vi "add.issue.vi"(0 "issues in":map{i32, T2}(c390), 1 "creator map in":T1(c390), 2 "Path":path, 5 "char map in":T3, 7 "concept map in":T3, 9 "story map in":T3, 11 "error in (no error)":errorcluster, 12 "team map in":T3) -> (3 "creator map out":T1(c390), 4 "issues out":map{i32, T2}(c390), 6 "char map out":T3, 8 "concept map out":T3, 10 "story map out":T3, 14 "team map out":T3, 15 "error out":errorcluster)   [LabVIEW 2024, in "manager_daemon.lvclass"]
uses:
  manager_daemon.lvclass
  type_defs/sub-map--map.ctl
  type_defs/SubData--cluster.ctl
  type_defs/IssueData--clustrer.ctl
  manager_daemon.lvclass/manager_daemon.ctl
  CV_Shared_Library/CV_Shared_Library.lvlib
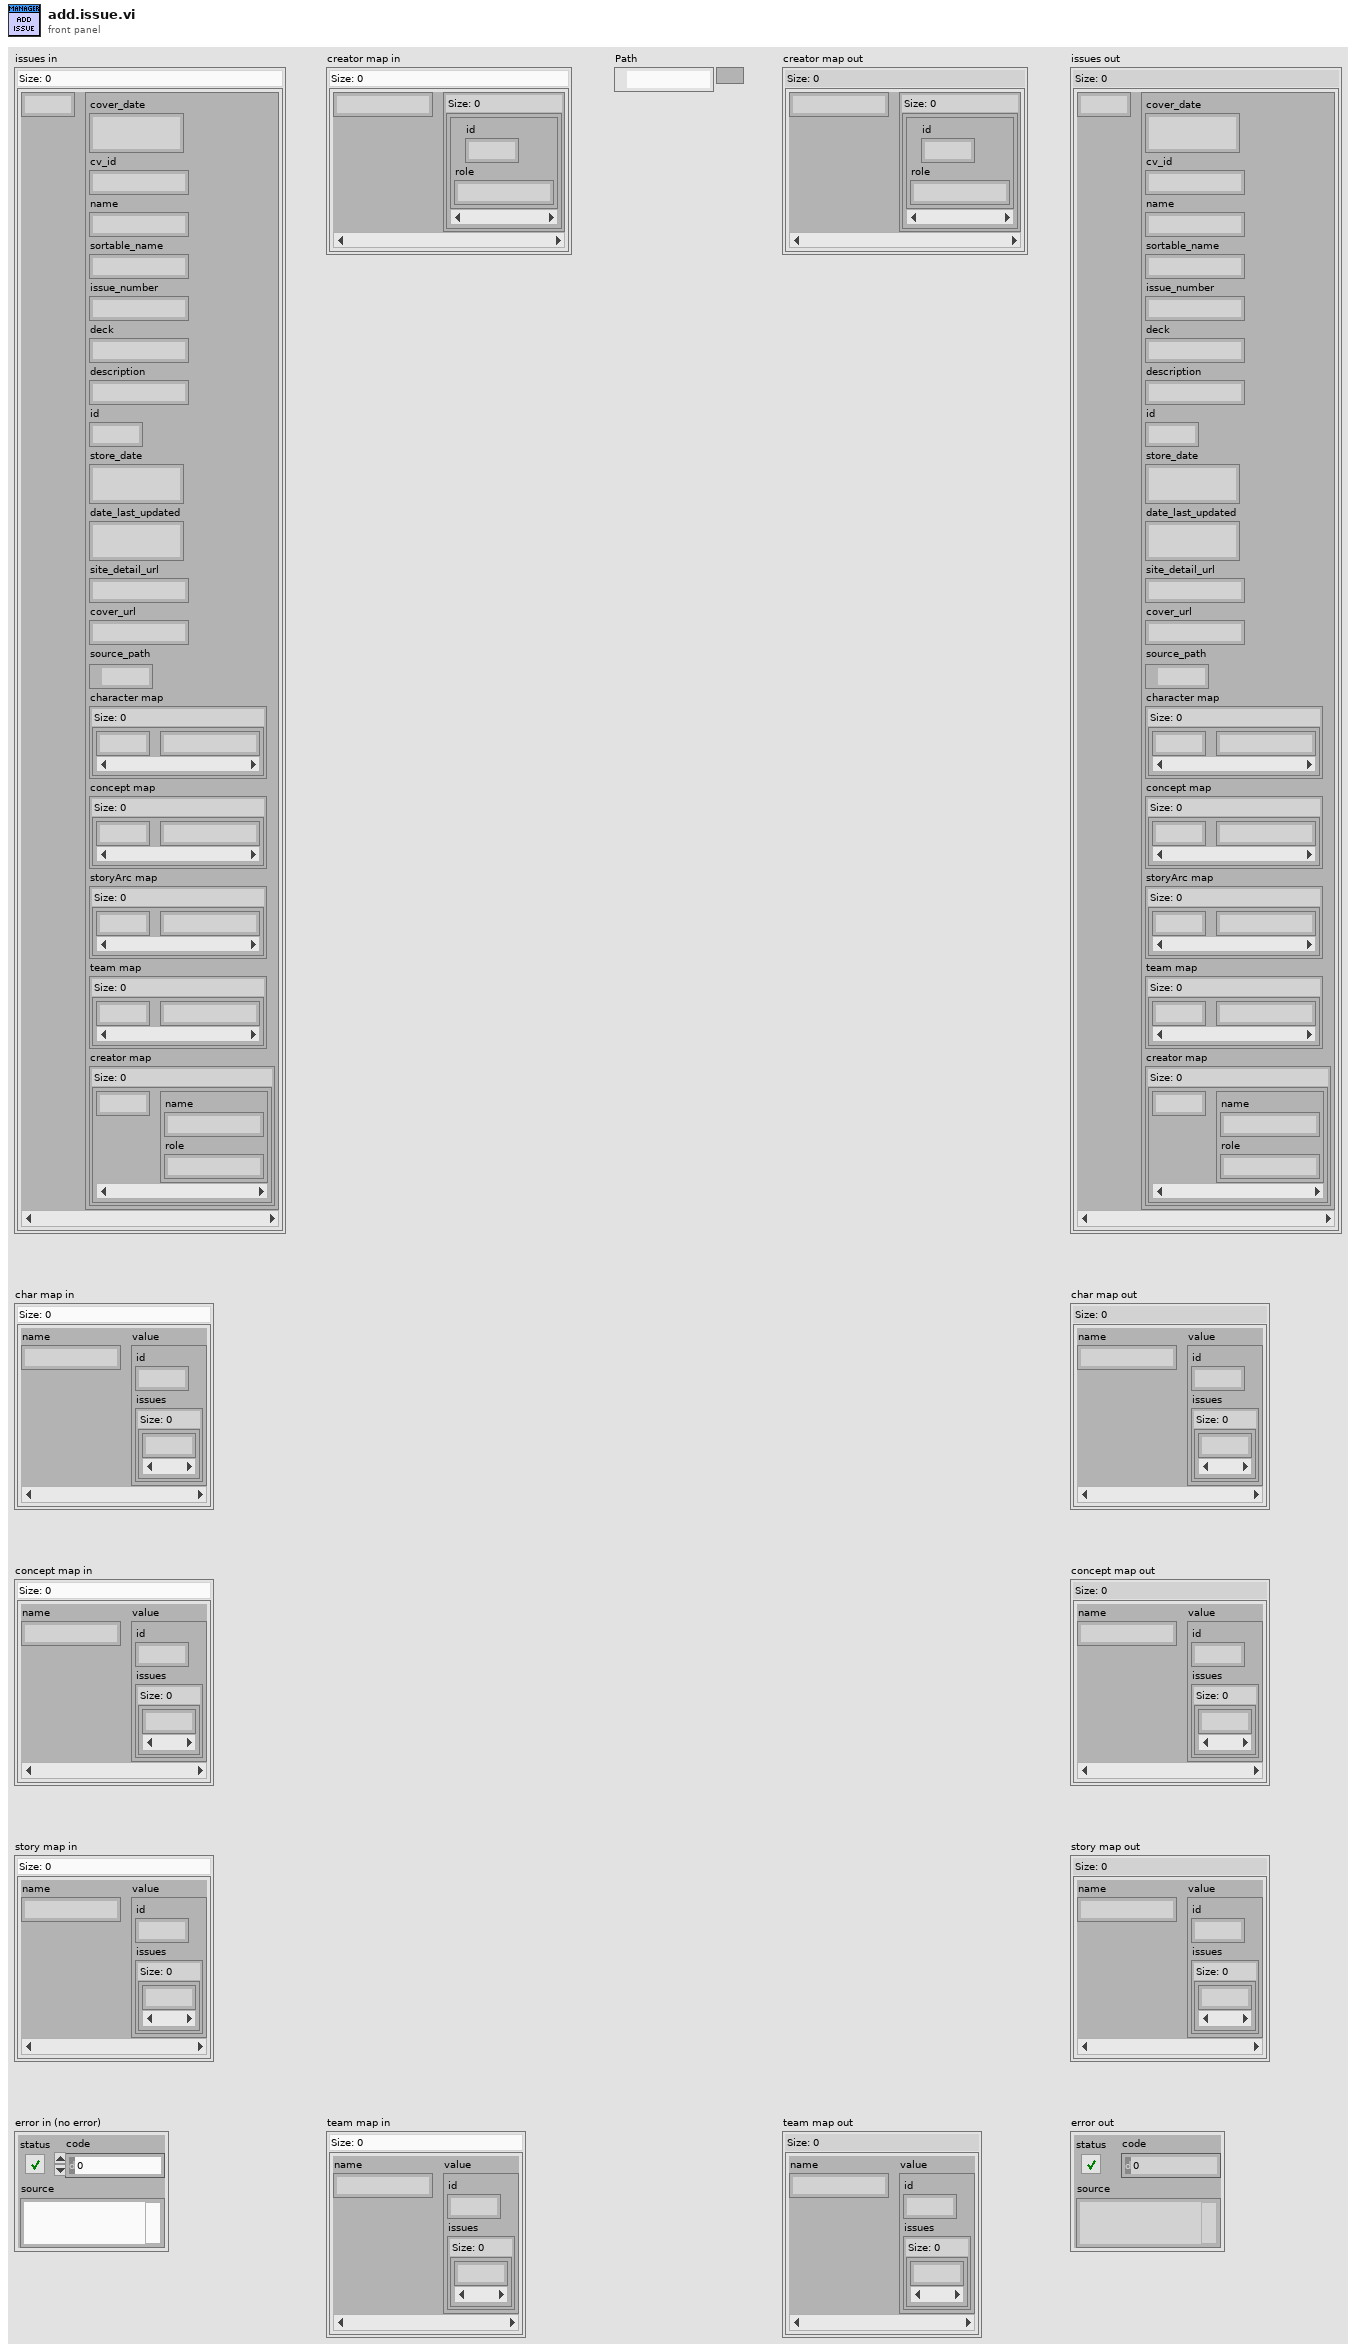
[diagram p1: front panel]
types:
  T1 = map{string, set{cluster{"id":i32, "role":string}}}
  T2 = typedef "manager_daemon.lvclass/IssueData--clustrer.ctl" = cluster{"cover_date":timestamp, "cv_id":string, "name":string, "sortable_name":string, "issue_number":string, "deck":string, "description":string, "id":i32, "store_date":timestamp, "date_last_updated":timestamp, "site_detail_url":string, "cover_url":string, "source_path":path, "character map":map{i32, string}, "concept map":map{i32, string}, "storyArc map":map{i32, string}, "team map":map{i32, string}, "creator map":map{i32, cluster{"name":string, "role":string}}}
  T3 = typedef "manager_daemon.lvclass/sub-map--map.ctl" = map{string, T4}
  T4 = typedef "manager_daemon.lvclass/SubData--cluster.ctl" = cluster{"id":i32, "issues":set{i32}}
  T5 = typedef "CV_RESTful_Lib.lvlib/local_issue--cluster.ctl" = cluster{"cover_date":timestamp, "id":i32, "cv_id":string, "name":string, "sortable_name":string, "issue_number":string, "deck":string, "description":string, "volume":T6, "store_date":timestamp, "date_last_updated":timestamp, "site_detail_url":string, "cover_url":string, "associated_images":T7[], "characters":T6[], "concepts":T6[], "creators":T8[], "storyArcs":T6[], "teams":T6[]}
  T6 = typedef "CV_RESTful_Lib.lvlib/cv_issue.generic_credit--cluster.ctl" = cluster{"id":i32, "name":string}
  T7 = typedef "CV_RESTful_Lib.lvlib/cv_issue.associated_image--cluster.ctl" = cluster{"original_url":string, "id":i32}
  T8 = typedef "CV_RESTful_Lib.lvlib/cv_issue.person_credit--cluster.ctl" = cluster{"id":i32, "name":string, "role":string}
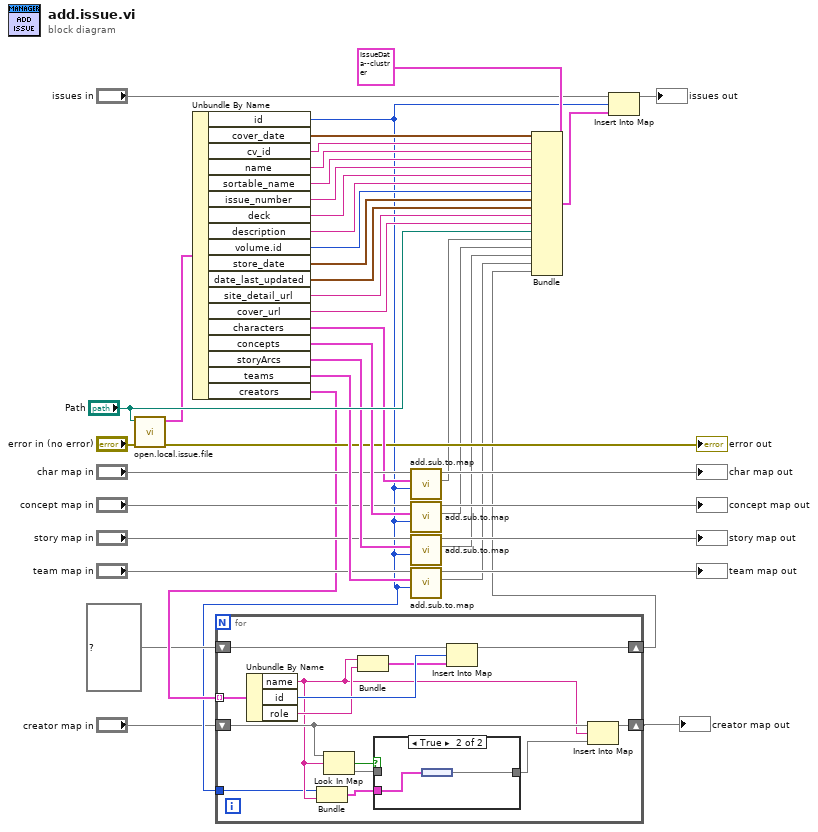
[diagram p0: block diagram]
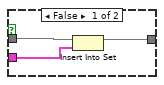
[diagram p2: hidden frame]
diagram:
  n1 = call "open.local.issue.file.vi"("error in (no error)"="error in (no error)", "volume json"="Path") -> ("error out"=→"error out":errorcluster, "issue"=w12:T5)  [unwired: 8 in]
  n2 = Unbundle By Name(w12) -> ("id"=w3:i32, "cover_date"=w13:timestamp, "cv_id"=w14:string, "name"=w15:string, "sortable_name"=w16:string, "issue_number"=w17:string, "deck"=w18:string, "description"=w19:string, "volume.id"=w20:i32, "store_date"=w21:timestamp, "date_last_updated"=w22:timestamp, "site_detail_url"=w23:string, "cover_url"=w24:string, "characters"=w29:T6[], "concepts"=w38:T6[], "storyArcs"=w39:T6[], "teams"=w40:T6[], "creators"=w6:T8[])
  n3 = for {
    tunnel: w6 -> [w56] mode=indexing
    shift-right: [w54] -> w1
    shift-left: "creator map in" -> [w52]
    tunnel: w3 -> [w44]
    shift-right: [w50] -> w4
    shift-left: map{i32, cluster{"name":string, "role":string}} {} ("map") -> [w51]
    n4 = Unbundle By Name(w56) -> ("name"=w45:string, "id"=w49:i32, "role"=w48:string)
    n5 = Bundle("id"=w44, "name"=w45) -> (w46:cluster{"id":i32, "name":string})  [unwired: 1 in]
    n6 = Look In Map(map=w52, key=w45) -> (key not found?=w55:bool, value=w53:set{cluster{"id":i32, "role":string}})  [unwired: 1 in]
    n7 = Bundle("name"=w45, "role"=w48) -> (w47:cluster{"name":string, "role":string})  [unwired: 1 in]
    n8 = case shown="True" w55 {
      tunnel: w46 -> [w59 w61]
      tunnel: w53 -> [w57 _]
      tunnel: [w58 w60] -> w43
      frame False {
        n9 = Insert Into Set(10:w59, 11:w57) -> (3:w58:set{cluster{"id":i32, "role":string}})  [unwired: 1 out]
      }
      frame True {
        n10 = node(w61) -> (w60:set{cluster{"id":i32, "name":string}})
      }
    }
    n11 = Insert Into Map(map in=w51, key=w49, value=w47) -> (map out=w50:map{i32, cluster{"name":string, "role":string}})  [unwired: 2 out]
    n12 = Insert Into Map(map in=w52, key=w45, value=w43) -> (map out=w54:T1)  [unwired: 2 out]
  }
  "creator map out" <- w1
  n13 = call "add.sub.to.map.vi"("id"=w3, "data"=w29, "map out"="char map in") -> ("issue map"=w10:map{i32, string}, "map out"=→"char map out":T3)  [unwired: 7 in]
  n14 = call "add.sub.to.map.vi"("id"=w3, "data"=w38, "map out"="concept map in") -> ("issue map"=w9:map{i32, string}, "map out"=→"concept map out":T3)  [unwired: 7 in]
  n15 = call "add.sub.to.map.vi"("id"=w3, "data"=w39, "map out"="story map in") -> ("issue map"=w8:map{i32, string}, "map out"=→"story map out":T3)  [unwired: 7 in]
  n16 = call "add.sub.to.map.vi"("id"=w3, "data"=w40, "map out"="team map in") -> ("issue map"=w7:map{i32, string}, "map out"=→"team map out":T3)  [unwired: 7 in]
  n17 = Bundle(cluster=T2 {"cover_date"=timestamp(0 s since 1904-01-01), "cv_id"="", "name"="", "sortable_name"="", "issue_number"="", "deck"="", "description"="", "id"=0, "store_date"=timestamp(0 s since 1904-01-01), "date_last_updated"=timestamp(0 s since 1904-01-01), "site_detail_url"="", "cover_url"="", "source_path"=path "", "character map"={}, "concept map"={}, "storyArc map"={}, "team map"={}, "creator map"={}} ("issue data"), "cover_date"=w13, "cv_id"=w14, "name"=w15, "sortable_name"=w16, "issue_number"=w17, "deck"=w18, "description"=w19, "id"=w20, "store_date"=w21, "date_last_updated"=w22, "site_detail_url"=w23, "cover_url"=w24, "source_path"="Path", "character map"=w10, "concept map"=w9, "storyArc map"=w8, "team map"=w7, "creator map"=w4) -> (w26:T2)
  n18 = Insert Into Map(map in="issues in", key=w3, value=w26) -> (map out=→"issues out":map{i32, T2})  [unwired: 2 out]
